vi "Frequency Measurements - Low Frequency with 1 Counter.vi"() -> ()   [LabVIEW 2009]
uses:
  <vilib>/DAQmx/create/channels.llb/DAQmx Create Channel (CI-Frequency).vi
  <vilib>/DAQmx/read.llb/DAQmx Read (Counter DBL 1Chan 1Samp).vi
panel:
  in  "stop":bool
  in  "counter":tag
  out "Frequency (Hz)":dbl format="%0.2f"
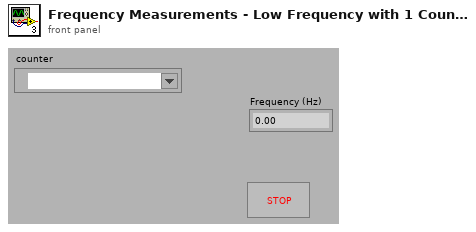
[diagram p1: front panel]
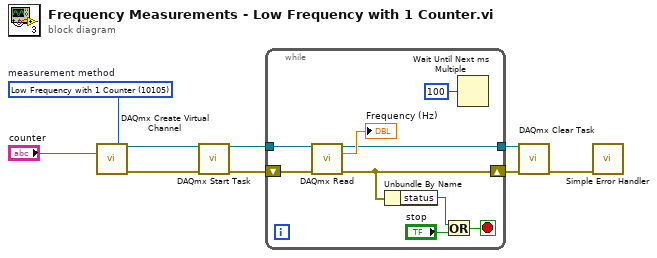
[diagram p0: block diagram]
diagram:
  w8 = 10105 items=["Low Frequency with 1 Counter"=10105, "High Frequency with 2 Counters"=10157, "Large Range with 2 Counters"=10205]  # measurement method
  n1 = call-poly <vilib>:"DAQmx Create Virtual Channel.vi"("measurement method"=w8, "counter"="counter") -> ("task out"=w7:refnum<k21>, "error out"=w5:errorcluster)  [unwired: 12 in]
  n2 = call <vilib>:"DAQmx Start Task.vi"("task/channels in"=w7, "error in"=w5) -> ("task out"=w6:refnum<k21>, "error out"=w4:errorcluster)  [unwired: 12 in]
  n3 = while {
    tunnel: w6 -> [w16]
    shift-right: [w15] -> w2
    shift-left: w4 -> [w17]
    tunnel: [w10] -> w3
    stop <- w14 stop-if-true
    n4 = call-poly <vilib>:"DAQmx Read.vi"("task/channels in"=w16, "error in"=w17) -> ("task out"=w10:refnum<k21>, "data"=→"Frequency (Hz)":dbl, "error out"=w15:errorcluster)  [unwired: 11 in]
    n5 = Unbundle By Name "Unbundle By Name"(w15) -> ("status"=w13:bool)
    n6 = Or(x=w13, y="stop") -> (x .or. y?=w14:bool)
    n7 = Wait Until Next ms Multiple(millisecond multiple=u32 100) -> ()  [unwired: 1 out]
  }
  n8 = call <vilib>:"DAQmx Clear Task.vi"("task in"=w3, "error in"=w2) -> ("error out"=w1:errorcluster)  [unwired: 13 in]
  n9 = call <vilib>:"Simple Error Handler.vi"("error in (no error)"=w1) -> ()  [unwired: 4 in, 5 out]
